vi "[FGV]BIOMETRICS.vi"(9 "Data in":sgl[](array[numeric]), 10 "Select":enum16{"READ", "WRITE"}(ring)) -> (1 "Data out":sgl[](array[numeric]))   [LabVIEW 2018]
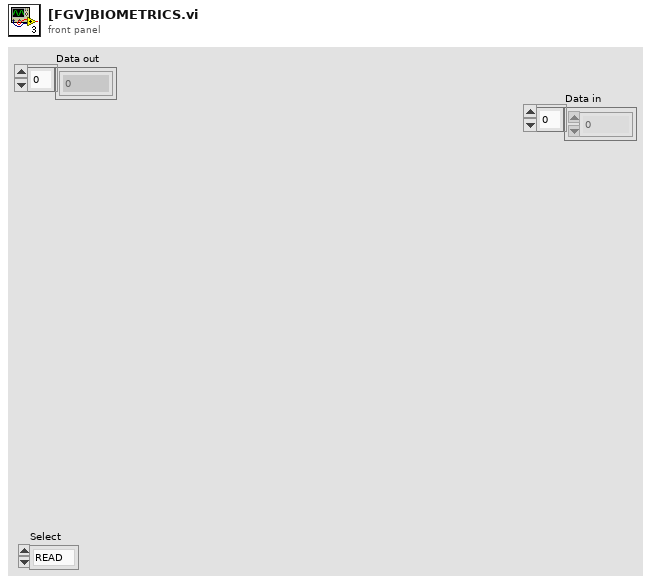
[diagram p1: front panel]
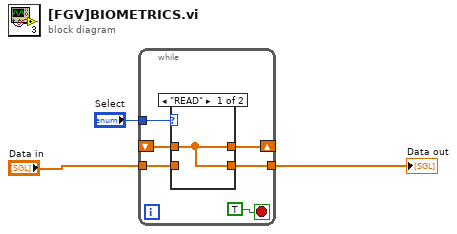
[diagram p0: block diagram]
diagram:
  n1 = while {
    tunnel: "Select" -> [w9]
    tunnel: [w8] -> w1
    shift-right: [w7] -> _
    shift-left: _ -> [w6]
    tunnel: "Data in" -> [w5]
    stop <- TRUE stop-if-true
    n2 = case shown="\"READ\"" w9 {
      tunnel: w6 -> [w10 _]
      tunnel: [w10 w11] -> w8
      tunnel: [w10 w11] -> w7
      tunnel: w5 -> [_ w11]
      frame "READ" {
      }
      frame "WRITE" {
      }
    }
  }
  "Data out" <- w1
